vi "Set File Read Only.vi"(2 "Make ReadOnly":bool, 3 "Path":path) -> (0 "Was found?":bool, 1 "Dup Path":path)   [LabVIEW 2012]
panel:
  # "ReadOnly"
  # "Writable"
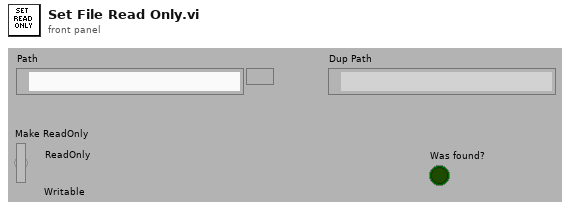
[diagram p1: front panel]
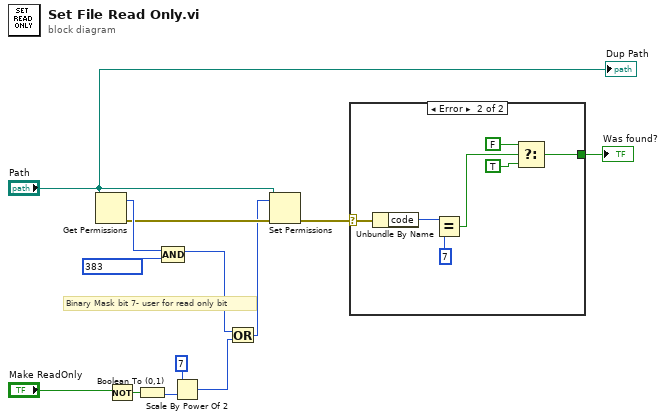
[diagram p0: block diagram]
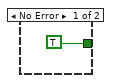
[diagram p2: hidden frame]
diagram:
  # "Binary Mask bit 7- user for read only bit"
  n1 = Get Permissions(11:"Path") -> (0:w4:errorcluster, 5:w11:i16)  [unwired: 1 in, 3 out]
  n2 = Not(x="Make ReadOnly") -> (.not. x?=w8:bool)
  n3 = Boolean To (0,1)(Boolean=w8) -> (0, 1=w7:i16)
  n4 = Compound Arithmetic op=AND(w11, 383) -> (w10:i32)
  n5 = Scale By Power Of 2(n=7, x=w7) -> (x*2^n=w5:i16)
  n6 = Or(x=w10, y=w5) -> (x .or. y?=w2:i32)
  n7 = Set Permissions(7:w2, 8:w4, 11:"Path") -> (0:w3:errorcluster)  [unwired: 3 out]
  n8 = case shown="Error" w3 {
    selector: w3 -> [_ w21]
    tunnel: [TRUE w17] -> w13
    frame No Error {
    }
    frame Error {
      n9 = Unbundle By Name(w21) -> ("code"=w20:i32)
      n10 = Equal?(x=w20, y=7) -> (x = y?=w16:bool)
      n11 = Select(t=FALSE, s=w16, f=TRUE) -> (s? t:f=w17:bool)
    }
  }
  "Was found?" <- w13
  "Dup Path" <- "Path"
